vi "Sync Channels.vi"() -> ()   [LabVIEW 2021]
uses:
  <vilib>/DAQmx/read.llb/DAQmx Read (Analog 1D Wfm NChan NSamp).vi
  <vilib>/DAQmx/create/channels.llb/DAQmx Create Channel (AI-Voltage-Basic).vi
  <vilib>/DAQmx/configure/timing.llb/DAQmx Timing (Sample Clock).vi
  <vilib>/DAQmx/configure/events/hardwareSignals.llb/DAQmx Export Signal (Most Signals).vi
  <vilib>/DAQmx/configure/trigger.llb/DAQmx Start Trigger (Digital Edge).vi
  <vilib>/DAQmx/miscellaneous.llb/DAQmx Fill In Error Info.vi
panel:
  out "Waveform Chart 2":waveform(dbl)[](graph)
  out "Waveform Chart":waveform(dbl)[](graph)
  in  "stop 2":bool
  out "task done? AI 2":bool
  out "task done? AI":bool
  in  "stop":bool
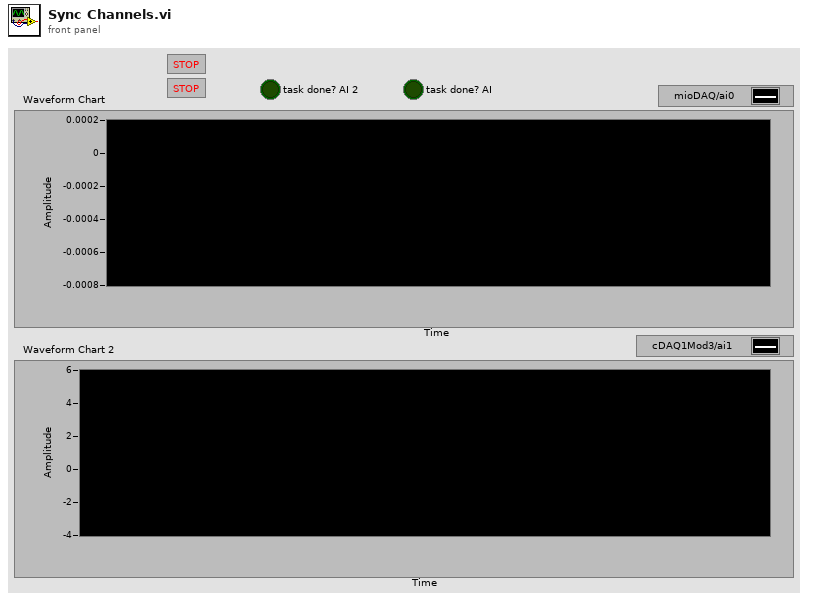
[diagram p1: front panel]
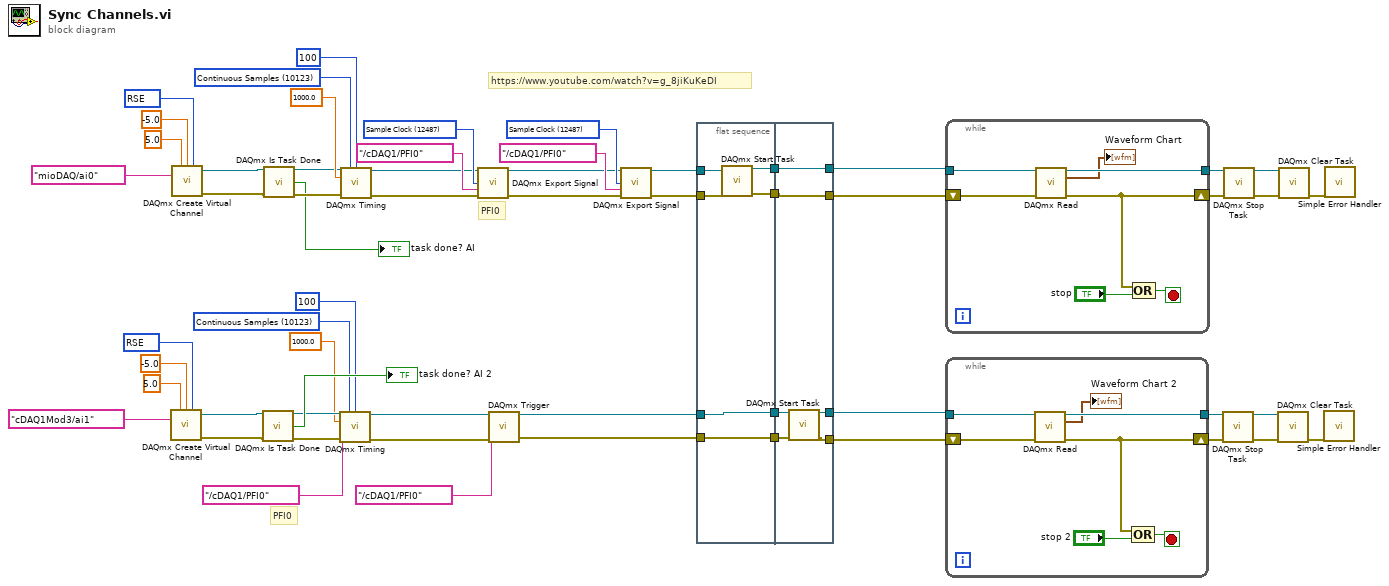
[diagram p0: block diagram]
diagram:
  w19 = 12487 items=["AI Convert Clock"=12484, "10MHz Reference Clock"=12536, "20MHz Timebase Clock"=12486, "Sample Clock"=12487, "Advance Trigger"=12488, "Reference Trigger"=12490, "Start Trigger"=12491, "Advance Complete Event"=12492, "AI Hold Complete Event"=12493, "Counter Output Event"=12494, "Change Detection Event"=12511, "Watchdog Timer Expired Event"=12512] ("signal")
  w24 = 12487 items=["AI Convert Clock"=12484, "10MHz Reference Clock"=12536, "20MHz Timebase Clock"=12486, "Sample Clock"=12487, "Advance Trigger"=12488, "Reference Trigger"=12490, "Start Trigger"=12491, "Advance Complete Event"=12492, "AI Hold Complete Event"=12493, "Counter Output Event"=12494, "Change Detection Event"=12511, "Watchdog Timer Expired Event"=12512] ("signal")
  w35 = 10083 items=["Default"=-1, "RSE"=10083, "NRSE"=10078, "Differential"=10106, "Pseudodifferential"=12529] ("input terminal configuration")
  w30 = 10123 items=["Finite Samples"=10178, "Continuous Samples"=10123, "Hardware Timed Single Point"=12522] ("sample mode")
  w48 = 10083 items=["Default"=-1, "RSE"=10083, "NRSE"=10078, "Differential"=10106, "Pseudodifferential"=12529] ("input terminal configuration")
  w53 = 10123 items=["Finite Samples"=10178, "Continuous Samples"=10123, "Hardware Timed Single Point"=12522] ("sample mode")
  # "PFI0"
  # "PFI0"
  # "https://www.youtube.com/watch?v=g_8jiKuKeDI"
  n1 = call-poly <vilib>:"DAQmx Create Virtual Channel.vi"("maximum value"=5.0, "minimum value"=-5.0, "input terminal configuration"=w35, "physical channels"=tag "cDAQ1Mod3/ai1") -> ("task out"=w37:refnum<k21>, "error out"=w38:errorcluster)  [unwired: 10 in]
  n2 = call-poly <vilib>:"DAQmx Create Virtual Channel.vi"("maximum value"=5.0, "minimum value"=-5.0, "input terminal configuration"=w48, "physical channels"=tag "mioDAQ/ai0") -> ("task out"=w46:refnum<k21>, "error out"=w45:errorcluster)  [unwired: 10 in]
  n3 = call <vilib>:"DAQmx Is Task Done.vi"("task/channels in"=w37, "error in"=w38) -> ("task out"=w40:refnum<k21>, "task done?"=→"task done? AI 2":bool, "error out"=w39:errorcluster)  [unwired: 11 in]
  n4 = call <vilib>:"DAQmx Is Task Done.vi"("task/channels in"=w46, "error in"=w45) -> ("task out"=w43:refnum<k21>, "task done?"=→"task done? AI":bool, "error out"=w44:errorcluster)  [unwired: 11 in]
  n5 = call-poly <vilib>:"DAQmx Timing.vi"("task/channels in"=w40, "sample mode"=w30, "samples per channel"=100, "rate"=1000.0, "source"=tag "/cDAQ1/PFI0", "error in"=w39) -> ("task out"=w13:refnum<k21>, "error out"=w14:errorcluster)  [unwired: 8 in]
  n6 = call-poly <vilib>:"DAQmx Timing.vi"("task/channels in"=w43, "sample mode"=w53, "samples per channel"=100, "rate"=1000.0, "error in"=w44) -> ("task out"=w22:refnum<k21>, "error out"=w21:errorcluster)  [unwired: 9 in]
  n7 = call-poly <vilib>:"DAQmx Export Signal.vi"("task/channels in"=w22, "signal"=w24, "output terminal"=tag "/cDAQ1/PFI0", "error in"=w21) -> ("task out"=w18:refnum<k21>, "error out"=w17:errorcluster)  [unwired: 10 in]
  n8 = call-poly <vilib>:"DAQmx Trigger.vi"("task/channels in"=w13, "source"=tag "/cDAQ1/PFI0", "error in"=w14) -> ("task out"=w4:refnum<k21>, "error out"=w2:errorcluster)  [unwired: 11 in]
  n9 = call-poly <vilib>:"DAQmx Export Signal.vi"("task/channels in"=w18, "signal"=w19, "output terminal"=tag "/cDAQ1/PFI0", "error in"=w17) -> ("task out"=w12:refnum<k21>, "error out"=w11:errorcluster)  [unwired: 10 in]
  n10 = flat-sequence {
    tunnel: w12 -> [w64]
    tunnel: w11 -> [w63]
    tunnel: [w62] -> w10
    tunnel: [w61] -> w8
    tunnel: w4 -> [w60]
    tunnel: [w60] -> w3
    tunnel: w2 -> [w59]
    tunnel: [w59] -> w1
    tunnel: w10 -> [w70]
    tunnel: [w70] -> w9
    tunnel: w8 -> [w69]
    tunnel: [w69] -> w7
    tunnel: [w68] -> w6
    tunnel: [w67] -> w5
    tunnel: w3 -> [w66]
    tunnel: w1 -> [w65]
    frame #0 {
      n11 = call <vilib>:"DAQmx Start Task.vi"("task/channels in"=w64, "error in"=w63) -> ("task out"=w62:refnum<k21>, "error out"=w61:errorcluster)  [unwired: 12 in]
    }
    frame #1 {
      n12 = call <vilib>:"DAQmx Start Task.vi"("task/channels in"=w66, "error in"=w65) -> ("task out"=w68:refnum<k21>, "error out"=w67:errorcluster)  [unwired: 12 in]
    }
  }
  n13 = while {
    shift-right: [w72] -> w58
    shift-left: w7 -> [w73]
    tunnel: w9 -> [w74]
    tunnel: [w75] -> w54
    stop <- w76 stop-if-true
    n14 = call-poly <vilib>:"DAQmx Read.vi"("task/channels in"=w74, "error in"=w73) -> ("task out"=w75:refnum<k21>, "data"=→"Waveform Chart":waveform(dbl)[], "error out"=w72:errorcluster)  [unwired: 11 in]
    n15 = Compound Arithmetic op=OR(w72, "stop") -> (w76:bool)
  }
  n16 = while {
    shift-right: [w79] -> w25
    shift-left: w5 -> [w80]
    tunnel: w6 -> [w81]
    tunnel: [w82] -> w29
    stop <- w83 stop-if-true
    n17 = call-poly <vilib>:"DAQmx Read.vi"("task/channels in"=w81, "error in"=w80) -> ("task out"=w82:refnum<k21>, "data"=→"Waveform Chart 2":waveform(dbl)[], "error out"=w79:errorcluster)  [unwired: 11 in]
    n18 = Compound Arithmetic op=OR(w79, "stop 2") -> (w83:bool)
  }
  n19 = call <vilib>:"DAQmx Stop Task.vi"("task/channels in"=w29, "error in"=w25) -> ("task out"=w27:refnum<k21>, "error out"=w26:errorcluster)  [unwired: 12 in]
  n20 = call <vilib>:"DAQmx Stop Task.vi"("task/channels in"=w54, "error in"=w58) -> ("task out"=w56:refnum<k21>, "error out"=w57:errorcluster)  [unwired: 12 in]
  n21 = call <vilib>:"DAQmx Clear Task.vi"("task in"=w27, "error in"=w26) -> ("error out"=w28:errorcluster)  [unwired: 13 in]
  n22 = call <vilib>:"DAQmx Clear Task.vi"("task in"=w56, "error in"=w57) -> ("error out"=w55:errorcluster)  [unwired: 13 in]
  n23 = call <vilib>:"Simple Error Handler.vi"("error in (no error)"=w28) -> ()  [unwired: 4 in, 5 out]
  n24 = call <vilib>:"Simple Error Handler.vi"("error in (no error)"=w55) -> ()  [unwired: 4 in, 5 out]
